vi "ButtonManualOverride.vi"(11 "Buttons":bool[](array[boolean])) -> ()   [LabVIEW 2014]
uses:
  Gantry/GantryGlobals.vi
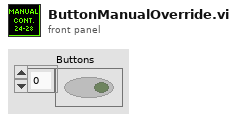
[diagram p1: front panel]
types:
  T1 = cluster{"proportional gain (Kc)":dbl, "integral time (Ti, min)":dbl, "derivative time (Td, min)":dbl}
  T2 = typedef "WPI_MotorControlDeviceRef.ctl" = cluster{"DeviceStatus":errorcluster, "Type":T3, "PWM":cluster{"Controller":T4, "PWM Channel":T5, "DeadBand":T6}, "CAN":cluster{"Device Number":u8, "Control Mode":T7, "Semaphore":T8, "Max Vout":dbl, "TalonSRX Control Mode":T9}, "Invert":bool, "TransformRef":T10, "InvTransformRef":T10}
  T3 = typedef "WPI_MotorControlType.ctl" = enum16{"PWM", "CAN", "CANTalonSRX"}
  T4 = typedef "FPGA_TypedefDigitalModule.ctl" = enum16{"Controller 1"}
  T5 = typedef "FPGA_DIOPWMChannel.ctl" = enum8{"PWM 0", "PWM 1", "PWM 2", "PWM 3", "PWM 4", "PWM 5", "PWM 6", "PWM 7", "PWM 8", "PWM 9", "PWM MXP 0", "PWM MXP 1", "PWM MXP 2", "PWM MXP 3", "PWM MXP 4", "PWM MXP 5", "PWM MXP 6", "PWM MXP 7", "PWM MXP 8", "PWM MXP 9", "Invalid"}
  T6 = typedef "WPI_PWMDeadband.ctl" = cluster{"Name":string, "maxPositivePwm":i32, "minPositivePwm":i32, "centerPwm":i32, "maxNegativePwm":i32, "minNegativePwm":i32, "angularRange":u16}
  T7 = typedef "WPI_CANJaguar_ControlMode.ctl" = enum8{"Percent VBus", "Current", "Speed", "Position", "Voltage"}
  T8 = typedef "Semaphore RefNum" = refnum<k1>
  T9 = typedef "WPI_CANTalonSRX_APIControlMode.ctl" = enum8{"Percent VBus", "Speed", "Position", "Slave", "Unchanged / Invalid"}
  T10 = typedef "WPI_PWMTransform_ConPane.ctl" = refnum<vi>
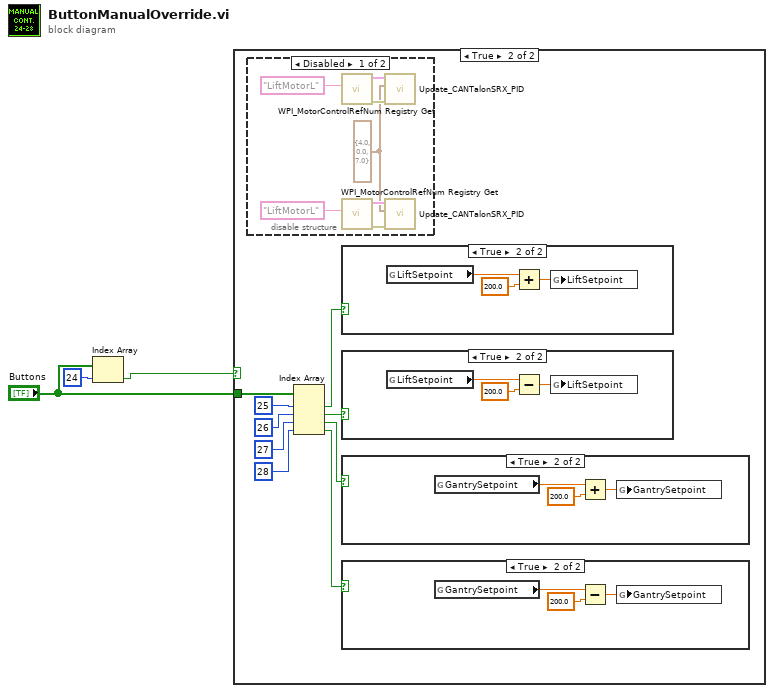
[diagram p0: block diagram]
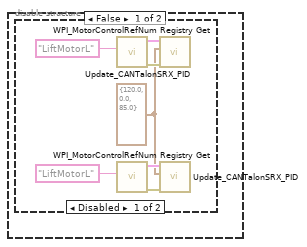
[diagram p2: hidden frame]
diagram:
  n1 = Index Array(array="Buttons", index=24) -> (element=w1:bool)
  n2 = case shown="True" w1 {
    tunnel: "Buttons" -> [_ w18]
    frame False {
      n3 = disable-structure shown="Disabled" {
        frame Disabled {
          w4 = T1 {"proportional gain (Kc)"=120.0, "integral time (Ti, min)"=0.0, "derivative time (Td, min)"=85.0} ("PID Gains")
          n4 = call <vilib>:"WPI_MotorControlRefNum Registry Get.vi"("refnum name"="LiftMotorL") -> ("error out"=w5:errorcluster, "MotorControlDevRef"=w6:T2)  [unwired: 9 in]
          n5 = call <vilib>:"WPI_MotorControlRefNum Registry Get.vi"("refnum name"="LiftMotorL") -> ("error out"=w8:errorcluster, "MotorControlDevRef"=w9:T2)  [unwired: 9 in]
          n6 = call "Update_CANTalonSRX_PID.vi"("error in (no error)"=w5, "PID Gains"=w4, "CAN Talon SRX Ref"=w6) -> ()  [unwired: 7 in, 2 out]
          n7 = call "Update_CANTalonSRX_PID.vi"("error in (no error)"=w8, "PID Gains"=w4, "CAN Talon SRX Ref"=w9) -> ()  [unwired: 7 in, 2 out]
        }
        frame Enabled {
        }
      }
    }
    frame True {
      n8 = disable-structure shown="Disabled" {
        frame Disabled {
          w20 = T1 {"proportional gain (Kc)"=4.0, "integral time (Ti, min)"=0.0, "derivative time (Td, min)"=7.0} ("PID Gains")
          n9 = call <vilib>:"WPI_MotorControlRefNum Registry Get.vi"("refnum name"="LiftMotorL") -> ("error out"=w21:errorcluster, "MotorControlDevRef"=w22:T2)  [unwired: 9 in]
          n10 = call <vilib>:"WPI_MotorControlRefNum Registry Get.vi"("refnum name"="LiftMotorL") -> ("error out"=w24:errorcluster, "MotorControlDevRef"=w25:T2)  [unwired: 9 in]
          n11 = call "Update_CANTalonSRX_PID.vi"("error in (no error)"=w21, "PID Gains"=w20, "CAN Talon SRX Ref"=w22) -> ()  [unwired: 7 in, 2 out]
          n12 = call "Update_CANTalonSRX_PID.vi"("error in (no error)"=w24, "PID Gains"=w20, "CAN Talon SRX Ref"=w25) -> ()  [unwired: 7 in, 2 out]
        }
        frame Enabled {
        }
      }
      n13 = Index Array(array=w18, index #1=25 ("index"), index #2=26 ("index"), index #3=27 ("index"), index #4=28 ("index")) -> (element #1=w17:bool, element #2=w13:bool, element #3=w12:bool, element #4=w11:bool)
      n14 = case shown="True" w17 {
        frame False {
        }
        frame True {
          n15 = global read "GantryGlobals.vi" "LiftSetpoint"() -> (w37:dbl)
          n16 = Add(x=w37, y=200.0) -> (x+y=w38:dbl)
          n17 = global write "GantryGlobals.vi" "LiftSetpoint"(w38) -> ()
        }
      }
      n18 = case shown="True" w13 {
        frame False {
        }
        frame True {
          n19 = global read "GantryGlobals.vi" "LiftSetpoint"() -> (w34:dbl)
          n20 = Subtract(x=w34, y=200.0) -> (x-y=w35:dbl)
          n21 = global write "GantryGlobals.vi" "LiftSetpoint"(w35) -> ()
        }
      }
      n22 = case shown="True" w12 {
        frame False {
        }
        frame True {
          n23 = global read "GantryGlobals.vi" "GantrySetpoint"() -> (w31:dbl)
          n24 = Add(x=w31, y=200.0) -> (x+y=w32:dbl)
          n25 = global write "GantryGlobals.vi" "GantrySetpoint"(w32) -> ()
        }
      }
      n26 = case shown="True" w11 {
        frame False {
        }
        frame True {
          n27 = global read "GantryGlobals.vi" "GantrySetpoint"() -> (w28:dbl)
          n28 = Subtract(x=w28, y=200.0) -> (x-y=w29:dbl)
          n29 = global write "GantryGlobals.vi" "GantrySetpoint"(w29) -> ()
        }
      }
    }
  }
